vi "Create.vi"(0 "Container":refnum<class "Container base.lvclass">, 11 "error in (no error)":errorcluster) -> (4 "LV MDI":refnum<class "LV MDI.lvclass">, 15 "error out":errorcluster)   [LabVIEW 2016, in "LV MDI.lvclass"]
doc: "Create reference for MDI Panel."
uses:
  LV MDI.lvclass
  Container/Container base/Container base.lvclass
  Document/Document base/Document.lvclass
  LV MDI.lvclass/LV MDI.ctl
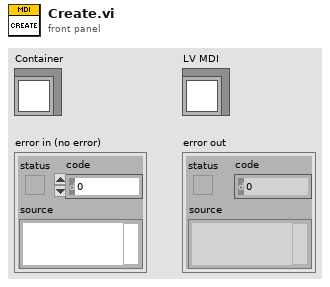
[diagram p1: front panel]
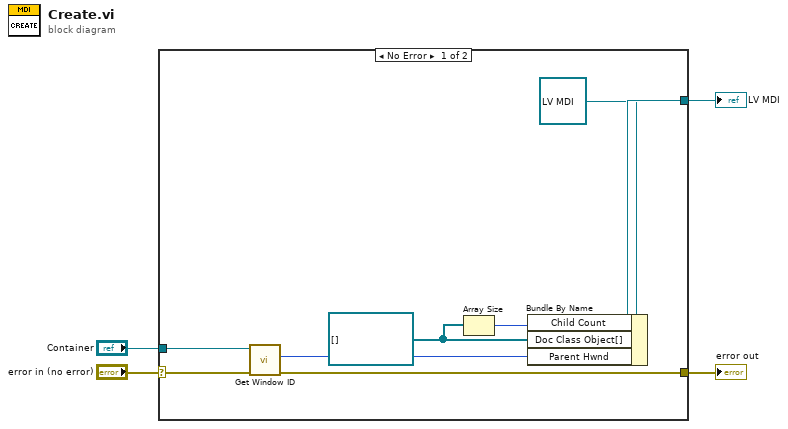
[diagram p0: block diagram]
diagram:
  n1 = case shown="No Error" "error in (no error)" {
    selector: "error in (no error)" -> [w9 w13]
    tunnel: [w8 w13] -> w3
    tunnel: [w12 _] -> w2
    tunnel: "Container" -> [w10 _]
    frame No Error {
      w6 = refnum<class "Document.lvclass">[] [] ("Doc Class Object[]")
      n2 = call-dynamic "Get Window ID.vi"("error in (no error)"=w9, "Container base in"=w10) -> ("error out"=w8:errorcluster, "HWND"=w7:i32)  [unwired: 7 in, 1 out]
      n3 = Array Size(array=w6) -> (size(s)=w5:i32)
      n4 = Bundle By Name(cluster=refnum<class "LV MDI.lvclass"> refnum ("LV MDI out"), "Child Count"=w5, "Doc Class Object[]"=w6, "Parent Hwnd"=w7) -> (w12:refnum<class "LV MDI.lvclass">)
    }
    frame Error {
    }
  }
  "error out" <- w3
  "LV MDI" <- w2
